vi "putHardpointStatus.vi"(8 "error in (no error)":errorcluster, 10 "TelemetryHardpointStatus":T1, 11 "Communicator in":refnum<class "Communicator.lvclass">) -> (0 "error out":errorcluster, 3 "Communicator out":refnum<class "Communicator.lvclass">)   [LabVIEW 2016, in "M1M3SupportCommunicator.lvlib" / "Communicator.lvclass"]
uses:
  Communicator.lvclass
  DataTypes/Topics/TelemetryHardpointStatus.ctl
  DataTypes/Topics/Parts/Timestamp.ctl
  DataTypes/Topics/M1M3SupportTopics.lvlib
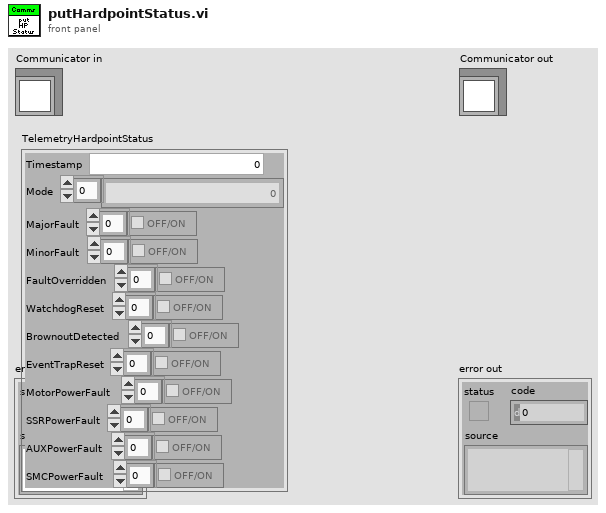
[diagram p1: front panel]
types:
  T1 = typedef "M1M3SupportTopics.lvlib/TelemetryHardpointStatus.ctl" = cluster{"Timestamp":T2, "Mode":u8[], "MajorFault":bool[], "MinorFault":bool[], "FaultOverridden":bool[], "WatchdogReset":bool[], "BrownoutDetected":bool[], "EventTrapReset":bool[], "MotorPowerFault":bool[], "SSRPowerFault":bool[], "AUXPowerFault":bool[], "SMCPowerFault":bool[]}
  T2 = typedef "M1M3SupportTopics.lvlib/Timestamp.ctl" = dbl
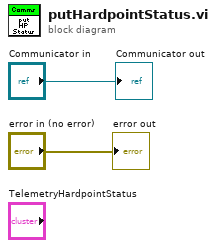
[diagram p0: block diagram]
diagram:
  "error out" <- "error in (no error)"
  "Communicator out" <- "Communicator in"
